vi "TENMA_Conf_On.vi"(8 "errin":errorcluster caption="entrée d'erreur (pas d'erreur)", 11 "Visa in tenma":refnum<visa-resource-name>) -> (0 "sortie d'erreur":errorcluster)   [LabVIEW 2020]
uses:
  <vilib>/Instr/_visa.llb/VISA Configure Serial Port (Instr).vi
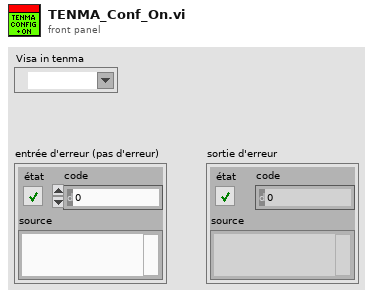
[diagram p1: front panel]
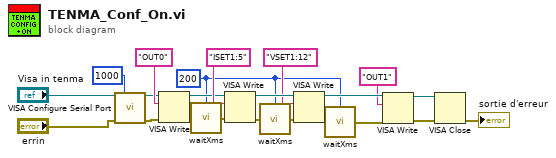
[diagram p0: block diagram]
diagram:
  w4 = u32 200 ("attente (ms)")
  n1 = call-poly "VISA Configure Serial Port"("VISA resource name"="Visa in tenma", "timeout (10sec)"=u32 1000, "error in (no error)"="errin") -> ("VISA resource name out"=w12:refnum<visa-resource-name>, "error out"=w13:errorcluster)  [unwired: 11 in]
  n2 = VISA Write(VISA resource name=w12, write buffer="OUT0" ("buffer d'écriture"), error in (no error)=w13) -> (VISA resource name out=w11:refnum<visa-resource-name>, error out=w10:errorcluster)  [unwired: 1 out]
  n3 = call <userlib>:"waitXms.vi"("attente (ms)"=w4, "errin"=w10) -> ("errout"=w9:errorcluster)  [unwired: 13 in]
  n4 = VISA Write(VISA resource name=w11, write buffer="ISET1:5" ("buffer d'écriture"), error in (no error)=w9) -> (VISA resource name out=w18:refnum<visa-resource-name>, error out=w8:errorcluster)  [unwired: 1 out]
  n5 = call <userlib>:"waitXms.vi"("attente (ms)"=w4, "errin"=w8) -> ("errout"=w7:errorcluster)  [unwired: 13 in]
  n6 = VISA Write(VISA resource name=w18, write buffer="VSET1:12" ("buffer d'écriture"), error in (no error)=w7) -> (VISA resource name out=w19:refnum<visa-resource-name>, error out=w5:errorcluster)  [unwired: 1 out]
  n7 = call <userlib>:"waitXms.vi"("attente (ms)"=w4, "errin"=w5) -> ("errout"=w6:errorcluster)  [unwired: 13 in]
  n8 = VISA Write(VISA resource name=w19, write buffer="OUT1" ("buffer d'écriture"), error in (no error)=w6) -> (VISA resource name out=w22:refnum<visa-resource-name>, error out=w21:errorcluster)  [unwired: 1 out]
  n9 = VISA Close(VISA resource name=w22, error in (no error)=w21) -> (error out=→"sortie d'erreur":errorcluster)
